vi "Generate Mappings.vi"() -> ()   [LabVIEW 2017]
panel:
  in  "file path":path
  in  "Starting Tx Channel":i32
  in  "Labels per Channel":i32=100
  in  "Number of Tx Channels":i32=16
  in  "dst base":string="Targets/Controller/Custom Devices/Ballard - Arinc-429/Outputs - Tx/"
  in  "src channel":string="Targets/Controller/Calculated Channels/Sine Wave 1 Hz"
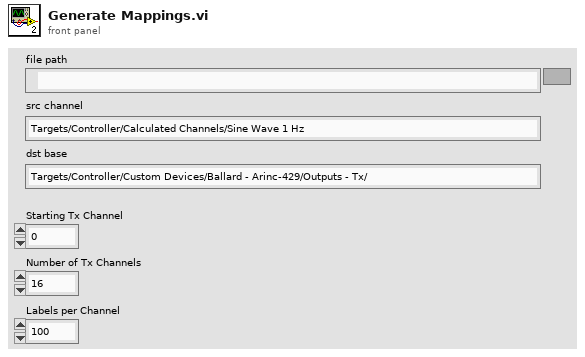
[diagram p1: front panel]
types:
  T1 = enum16{"open", "replace", "create", "open or create", "replace or create", "replace or create with confirmation"}
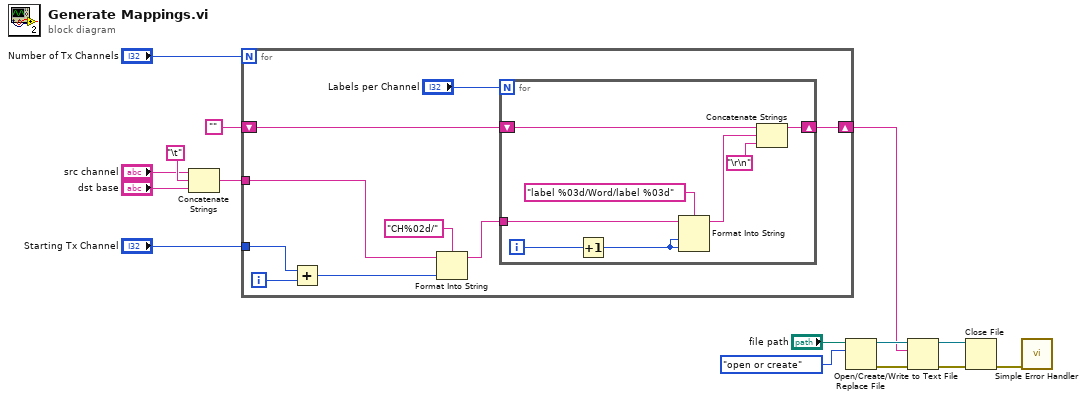
[diagram p0: block diagram]
diagram:
  n1 = Concatenate Strings("src channel", "\t", "dst base") -> (w10:string)
  n2 = for {
    N: "Number of Tx Channels" -> [_]
    shift-right: [w16] -> w4
    shift-left: "" -> [w17]
    tunnel: w10 -> [w21]
    tunnel: "Starting Tx Channel" -> [w20]
    i -> [w19]
    n3 = Add(x=w20, y=w19) -> (x+y=w18:i32)
    n4 = Format Into String(format string="CH%02d/", initial string=w21, w18) -> (resulting string=w22:string)  [unwired: 1 in, 1 out]
    n5 = for {
      N: "Labels per Channel" -> [_]
      tunnel: w22 -> [w30]
      shift-right: [w26] -> w16
      shift-left: w17 -> [w28]
      i -> [w31]
      n6 = Increment(x=w31) -> (x+1=w29:i32)
      n7 = Format Into String(format string="label %03d/Word/label %03d", initial string=w30, w29, w29) -> (resulting string=w27:string)  [unwired: 1 in, 1 out]
      n8 = Concatenate Strings(w28, w27, "\r\n") -> (w26:string)
    }
  }
  n9 = Open/Create/Replace File(file path (use dialog)="file path", operation (0:open)=T1."open or create") -> (refnum out=w6:refnum<file>, error out=w5:errorcluster)  [unwired: 4 in, 1 out]
  n10 = Write to Text File(file (use dialog)=w6, text=w4, error in=w5) -> (refnum out=w3:refnum<file>, error out=w2:errorcluster)  [unwired: 1 in, 1 out]
  n11 = Close File(refnum=w3, error in=w2) -> (error out=w1:errorcluster)  [unwired: 1 out]
  n12 = call <vilib>:"Simple Error Handler.vi"("error in (no error)"=w1) -> ()  [unwired: 4 in, 5 out]
